vi "Todas_Coincidencias_3_detectores.vi"() -> ()   [LabVIEW 2010]
uses:
  <vilib>/Instr/_visa.llb/VISA Configure Serial Port (Instr).vi
  <vilib>/Utility/file.llb/Write To Spreadsheet File (string).vi
panel:
  in  "Esperando Cuentas":bool
  in  "# Ventanas\na correr":i32=1
  out "# Ventana\nactual":i32=1
  out "Finalizado":bool=TRUE
  in  "INICIAR":bool
  out "Listo":bool=TRUE
  out "Tiempo \nTranscurrido (s)":i32=1
  in  "Config_Tiempo":bool
  in  "Tiempo de la ventana":i32=100
  in  "Unidades de tiempo":u16(ring) items=["(x10)ns", "us", "ms"]
  in  "Error Bytes,":bool
  in  "Guardar":bool
  in  "file path (dialog if empty)":path
  out "D123":u64=5
  out "D3":u64=1
  out "D2":u64=5
  out "D1":u64=10
  out "D23":u64=3
  out "D13":u64=5
  out "D12":u64=10
  out "Lectura":string
  in  "stop":bool
  out "Error":errorcluster
  in  "Puerto USB":refnum<visa-resource-name>="COM20"
  # "Unidad de conteo de coincidencias"
  # "johny.jaramillo@udea.edu.co"
  # "daniel.estrada1@udea.edu.co"
  # "Coincidencia \ntriple"
  # "Detectores \nIndividuales"
  # "Coincidencias \ndobles"
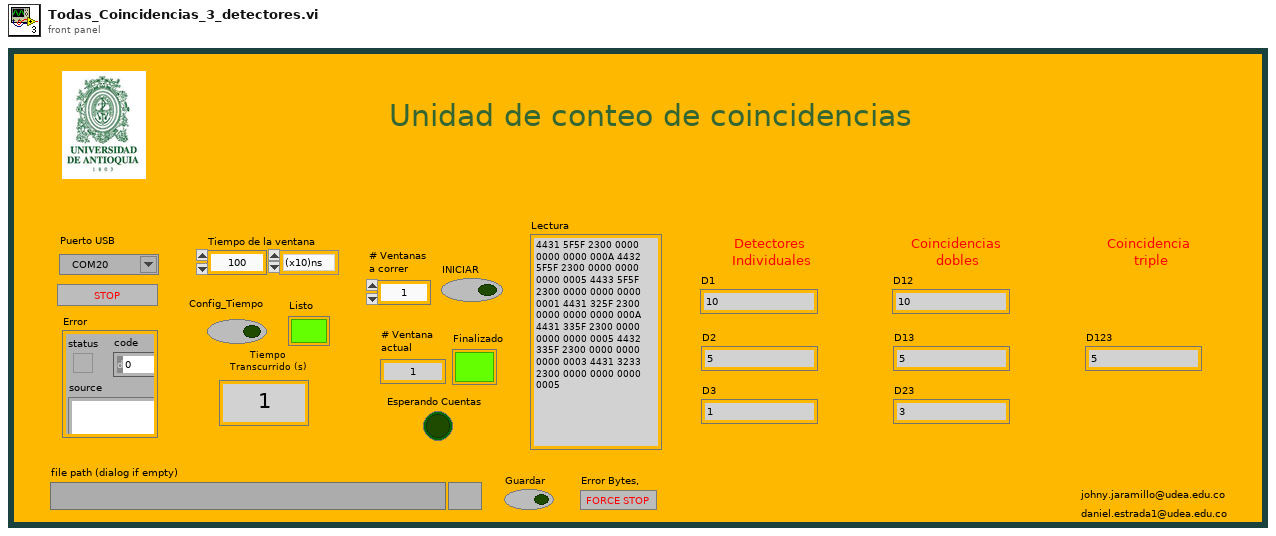
[diagram p1: front panel]
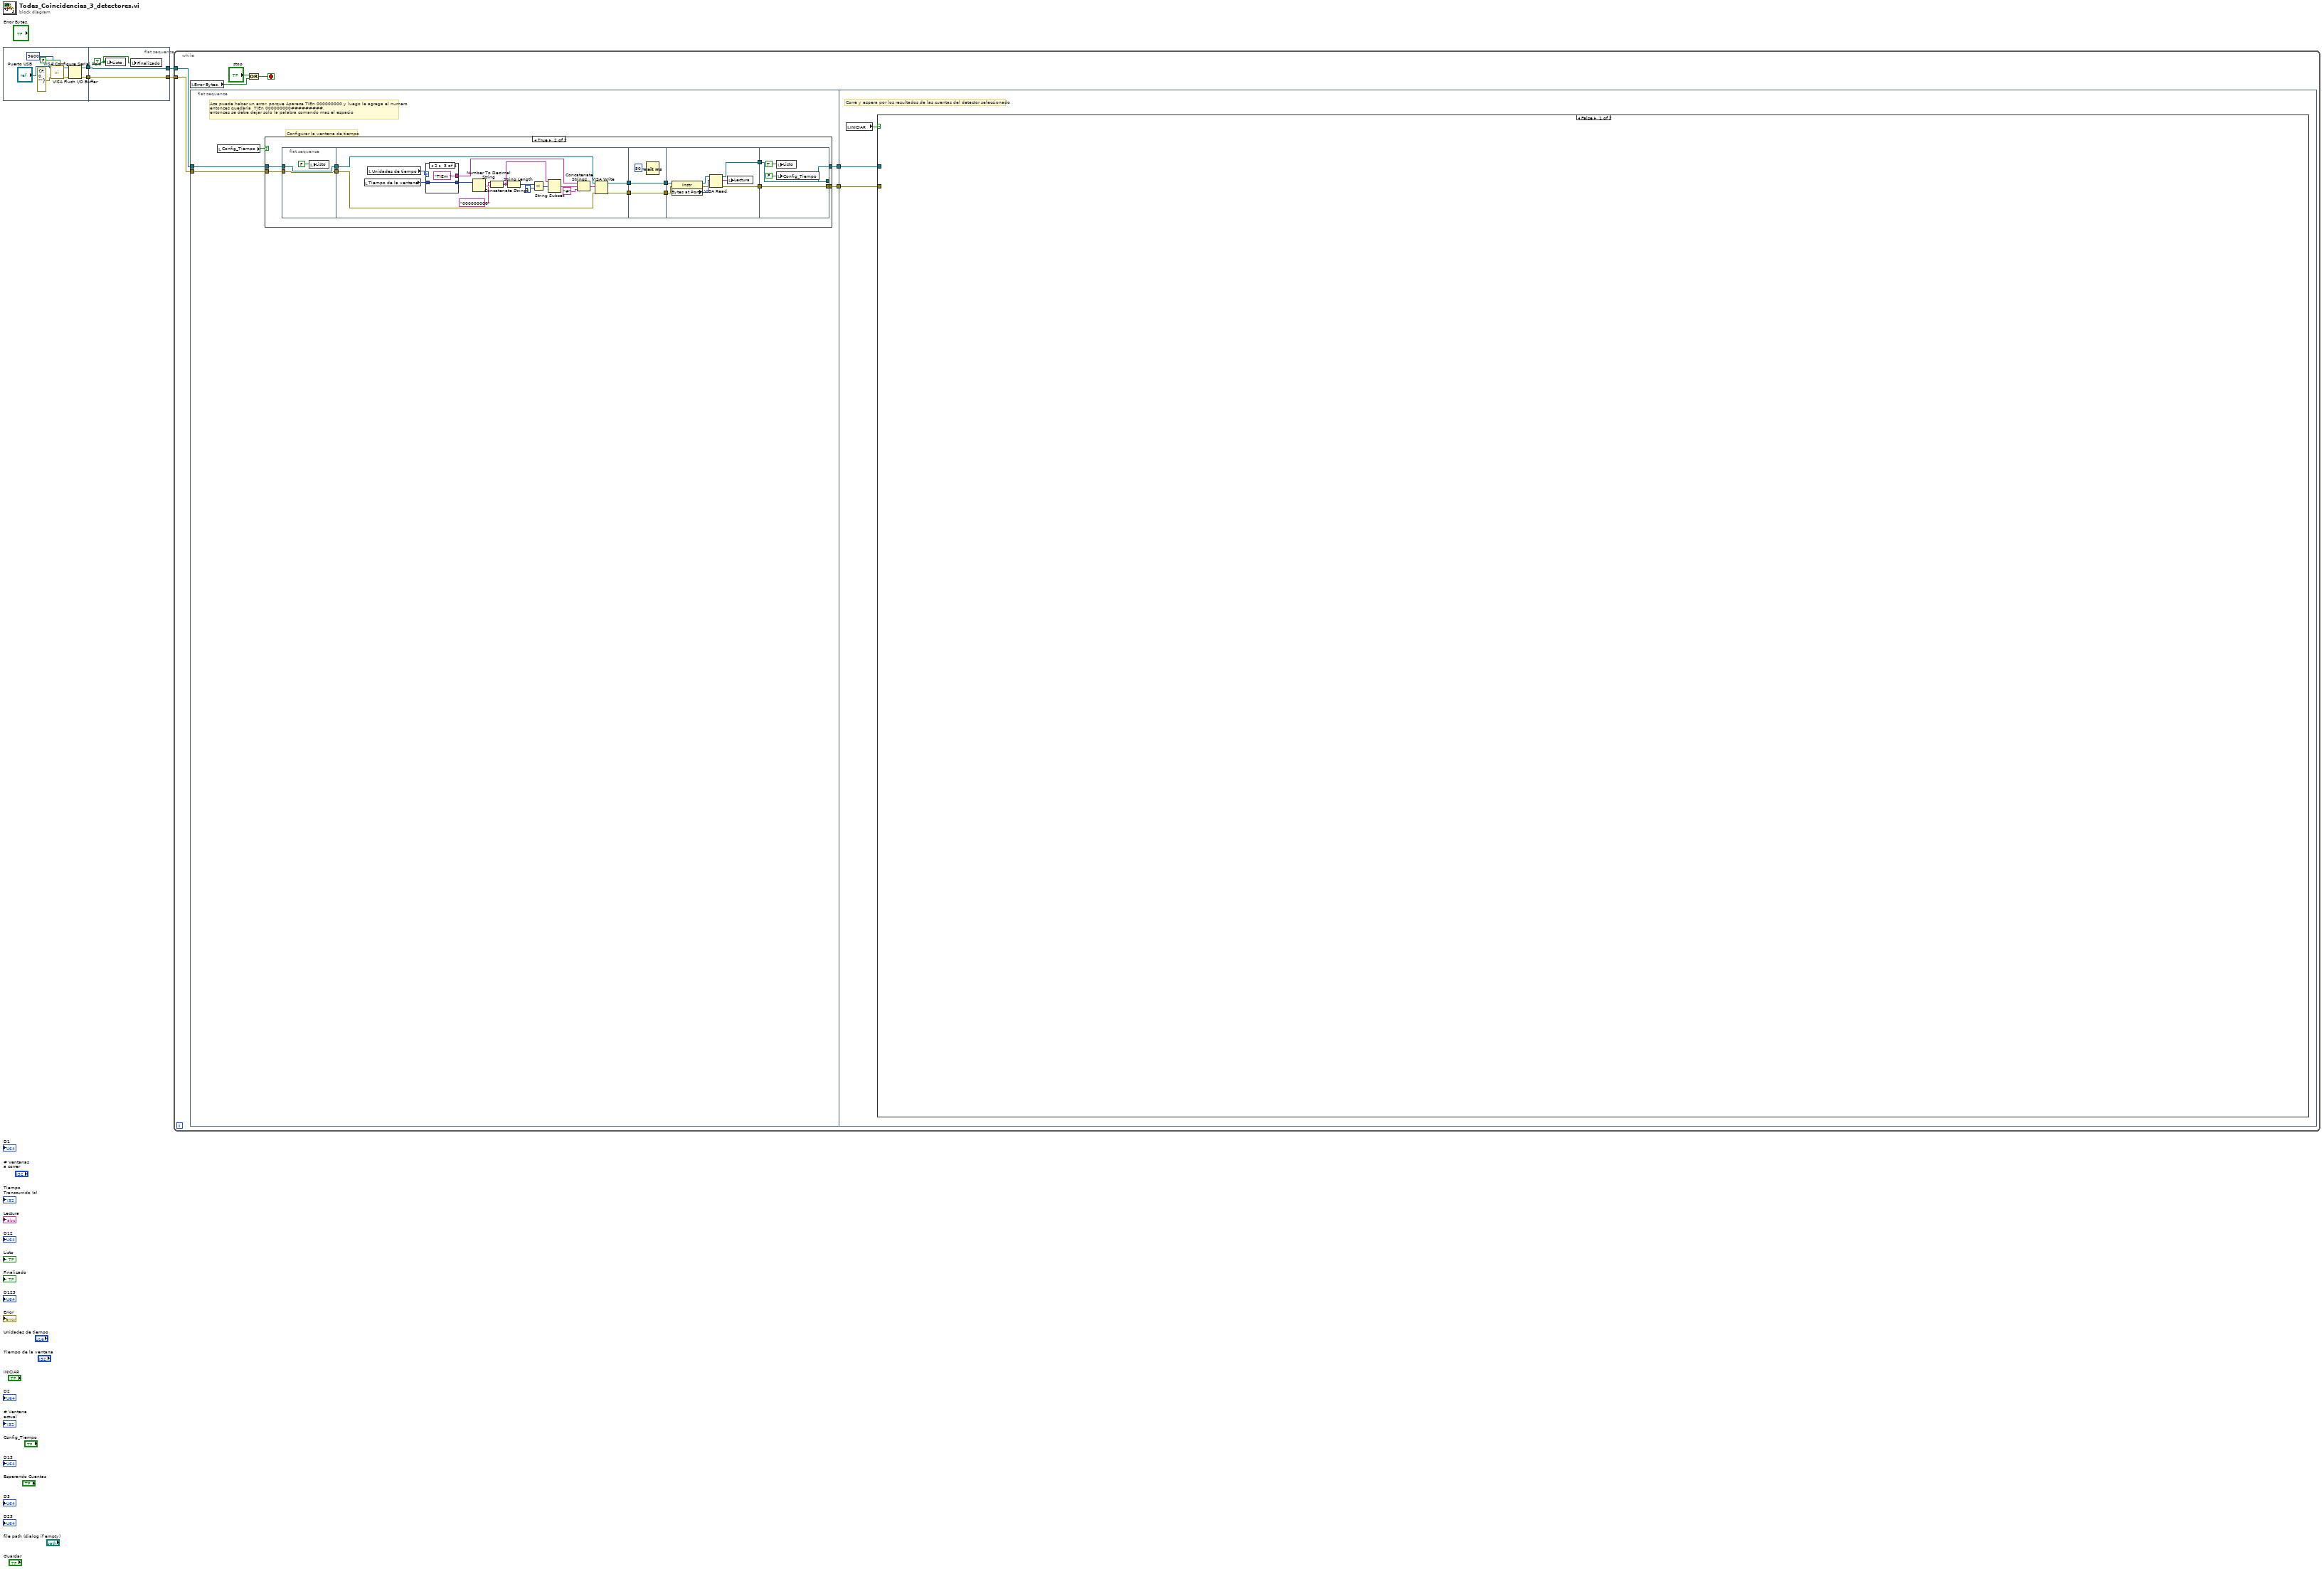
[diagram p0: block diagram]
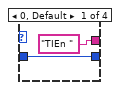
[diagram p3: hidden frame]
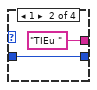
[diagram p4: hidden frame]
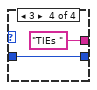
[diagram p5: hidden frame]
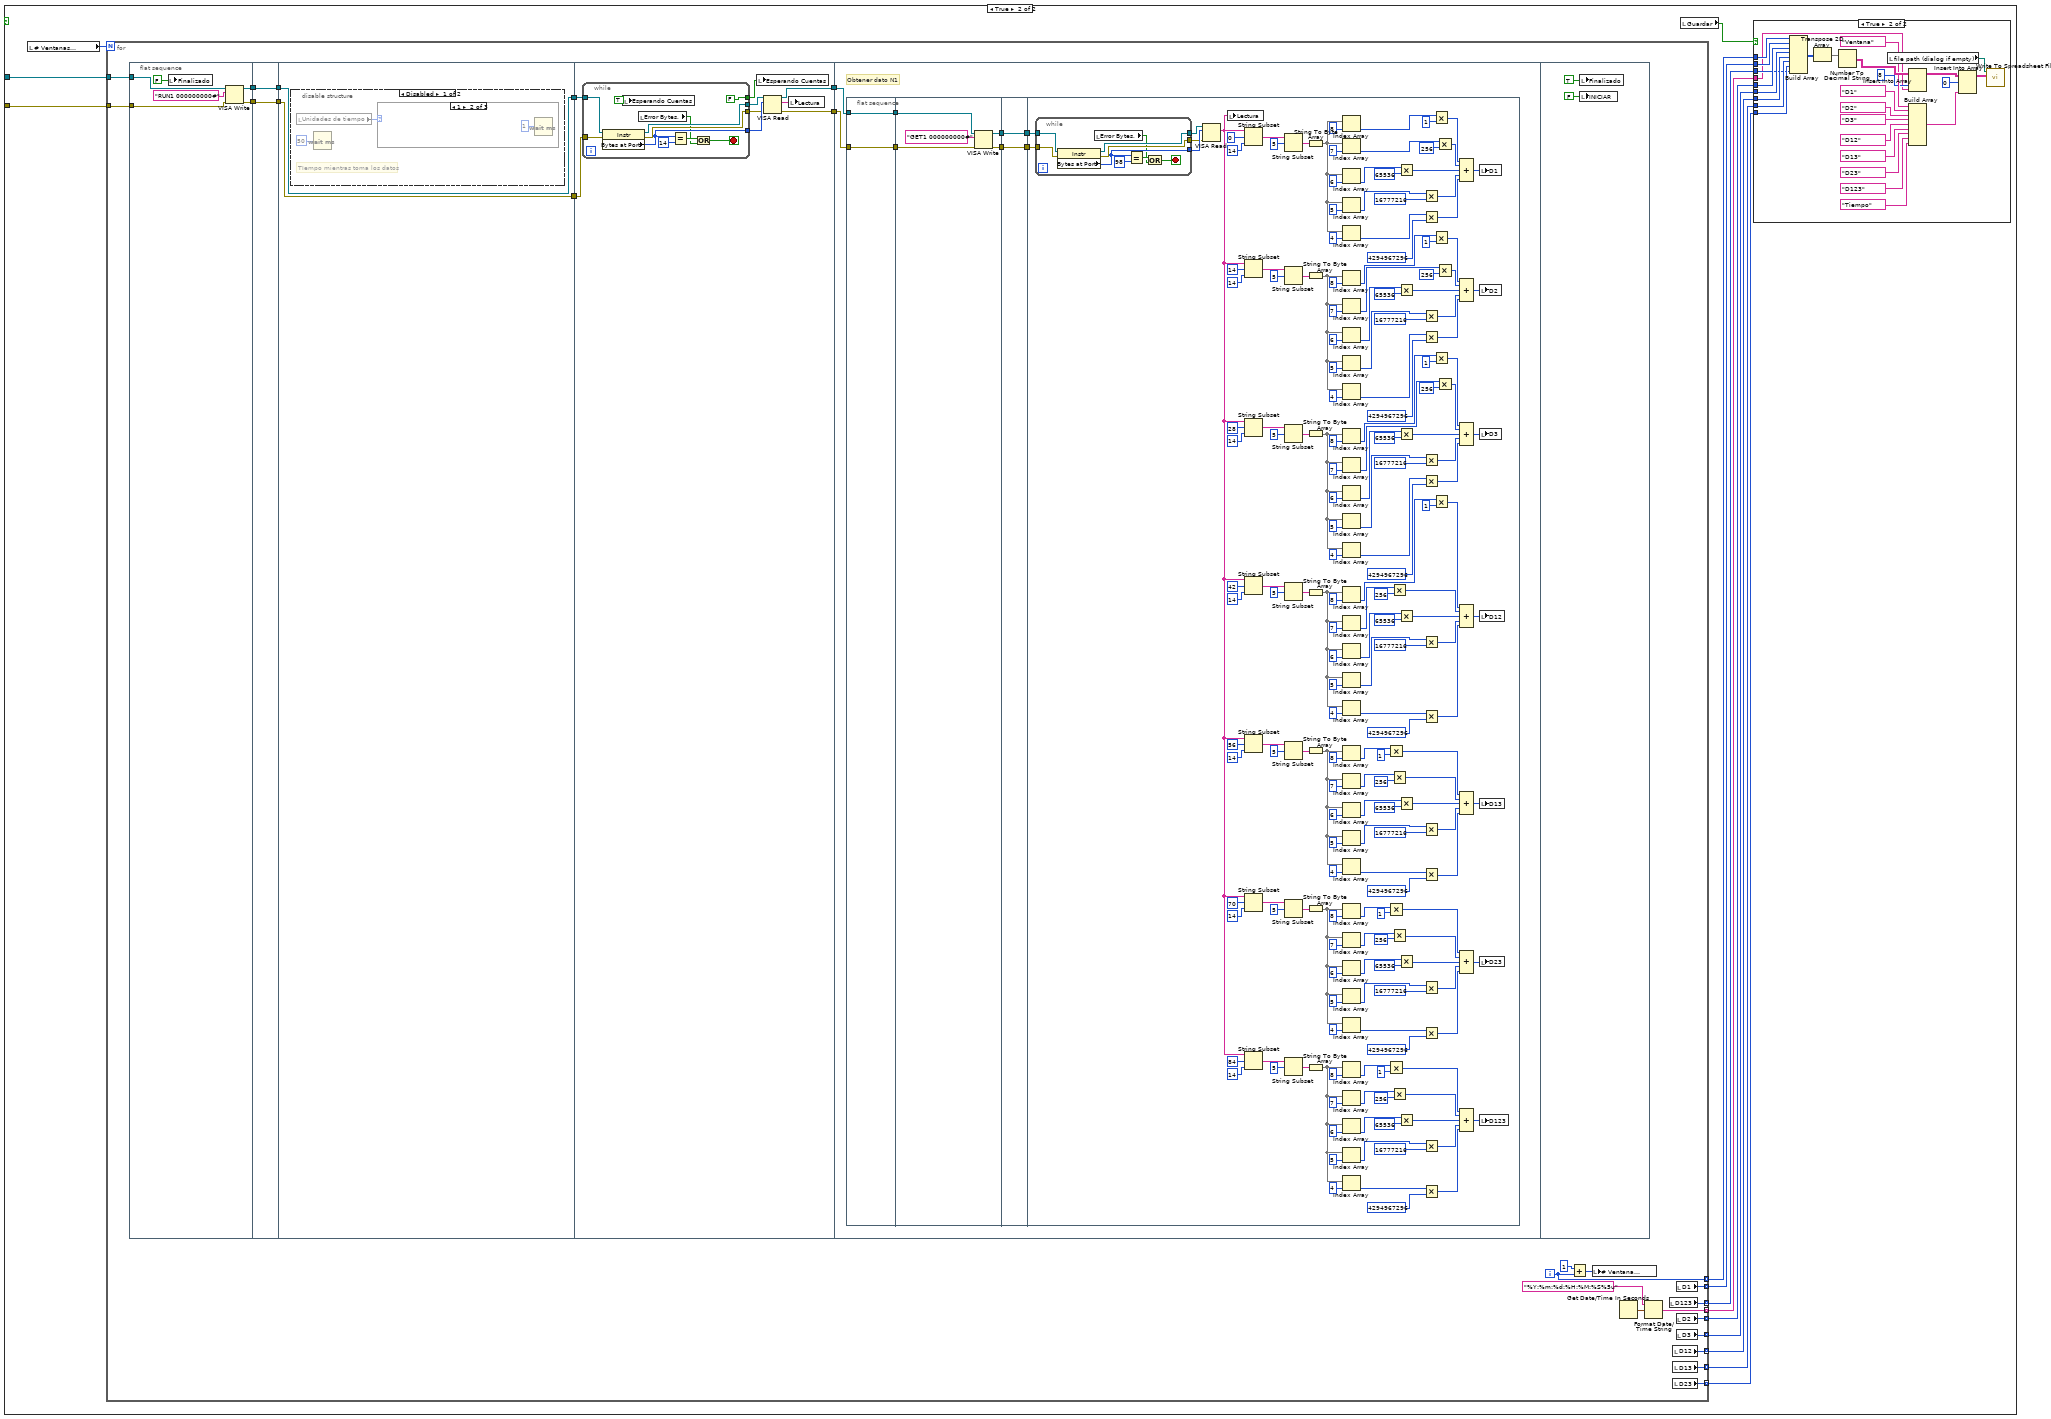
[diagram p6: hidden frame]
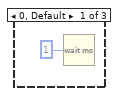
[diagram p8: hidden frame]
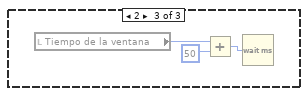
[diagram p9: hidden frame]
diagram:
  n1 = flat-sequence {
    tunnel: [w9] -> w4
    tunnel: [w8] -> w3
    tunnel: w4 -> [w14]
    tunnel: w3 -> [w13]
    tunnel: [w14] -> w2
    tunnel: [w13] -> w1
    frame #0 {
      n2 = call-poly "VISA Configure Serial Port"("VISA resource name"="Puerto USB", "Enable Termination\nChar (T)"=FALSE ("Enable Termination\nChar (T)"), "baud rate (9600)"=u32 9600, "error in (no error)"=errorcluster {"status"=FALSE, "code"=0, "source"=""}) -> ("VISA resource name out"=w7:refnum<visa-resource-name>, "error out"=w12:errorcluster)  [unwired: 10 in]
      n3 = VISA Flush I/O Buffer(VISA resource name=w7, error in (no error)=w12) -> (VISA resource name out=w9:refnum<visa-resource-name>, error out=w8:errorcluster)  [unwired: 1 in]
    }
    frame #1 {
      w15 = TRUE ("T. Done")
      n4 = local write "Listo"(w15) -> ()
      n5 = local write "Finalizado"(w15) -> ()
    }
  }
  n6 = while {
    tunnel: w2 -> [w20]
    tunnel: w1 -> [w19]
    stop <- w16 stop-if-true
    n7 = local read "Error Bytes,"() -> (w17:bool)
    n8 = flat-sequence {
      tunnel: [w26] -> w22
      tunnel: [w25] -> w21
      tunnel: w20 -> [w24]
      tunnel: w19 -> [w23]
      tunnel: w22 -> [w86]
      tunnel: w21 -> [w85]
      frame #0 {
        # "Aca puede haber un error, porque Aparece TIEn 000000000 y luego le agrega el numero\nentonces quedaria  TIEn 000000000#########,\nentonces se debe dejar solo la palabra comando mas el espacio"
        # "Configurar la ventana de tiempo"
        n9 = local read "Config_Tiempo"() -> (w27:bool)
        n10 = case shown="True" w27 {
          tunnel: [w29 w39] -> w26
          tunnel: [w28 w38] -> w25
          tunnel: w24 -> [w29 w41]
          tunnel: w23 -> [w28 w40]
          frame False {
          }
          frame True {
            n11 = flat-sequence {
              tunnel: w40 -> [w42]
              tunnel: w41 -> [w43]
              tunnel: [w43] -> w31
              tunnel: [w42] -> w30
              tunnel: [w59] -> w37
              tunnel: [w58] -> w35
              tunnel: w31 -> [w61]
              tunnel: w30 -> [w60]
              tunnel: w37 -> [w72]
              tunnel: [w72] -> w36
              tunnel: w35 -> [w71]
              tunnel: [w71] -> w34
              tunnel: w36 -> [w78]
              tunnel: w34 -> [w77]
              tunnel: [w75] -> w33
              tunnel: [w76] -> w32
              tunnel: [w83] -> w39
              tunnel: [w84] -> w38
              tunnel: w33 -> [w84]
              tunnel: w32 -> [w83]
              frame #0 {
                n12 = local write "Listo"(FALSE ("T. Done")) -> ()
              }
              frame #1 {
                n13 = local read "Tiempo de la ventana"() -> (w50:i32)
                n14 = local read "Unidades de tiempo"() -> (w51:u16)
                n15 = case shown="2" w51 {
                  tunnel: ["TIEn " ("string") "TIEu " ("string") "TIEm " ("string") "TIEs " ("string")] -> w57
                  tunnel: w50 -> [w62 w64 w66 w68]
                  tunnel: [w62 w64 w66 w68] -> w49
                  frame 0, Default {
                  }
                  frame 1 {
                  }
                  frame 2 {
                  }
                  frame 3 {
                  }
                }
                n16 = Number To Decimal String(number=w49) -> (decimal integer string=w53:string)  [unwired: 1 in]
                n17 = Concatenate Strings("000000000" ("string"), w53) -> (w54:string)
                n18 = String Length(string=w54) -> (length=w55:i32)
                n19 = Subtract(x=w55, y=9) -> (x-y=w46:i32)
                n20 = String Subset(string=w54, offset (0)=w46) -> (substring=w48:string)  [unwired: 1 in]
                n21 = Concatenate Strings(w57, w48, "#") -> (w45:string)
                n22 = VISA Write(VISA resource name=w61, write buffer=w45, error in (no error)=w60) -> (VISA resource name out=w59:refnum<visa-resource-name>, error out=w58:errorcluster)  [unwired: 1 out]
              }
              frame #2 {
                n23 = Wait (ms)(milliseconds to wait=u32 50) -> ()  [unwired: 1 out]
              }
              frame #3 {
                n24 = property class="Instr"(reference=w78, error in=w77) -> (reference out=w80:refnum<visa-resource-name>, error out=w74:errorcluster, "Bytes at Port"=w79:u32)
                n25 = VISA Read(VISA resource name=w80, byte count=w79, error in (no error)=w74) -> (VISA resource name out=w76:refnum<visa-resource-name>, read buffer=w73:string, error out=w75:errorcluster)  [unwired: 1 out]
                n26 = local write "Lectura"(w73) -> ()
              }
              frame #4 {
                n27 = local write "Listo"(TRUE ("T. Done")) -> ()
                n28 = local write "Config_Tiempo"(FALSE ("Config_Módulo")) -> ()
              }
            }
          }
        }
      }
      frame #1 {
        # "Corre y espera por los resultados de las cuentas del detector seleccionado"
        n29 = local read "INICIAR"() -> (w87:bool)
        n30 = case shown="False" w87 {
          tunnel: w86 -> [_ w100]
          tunnel: w85 -> [_ w99]
          frame False {
          }
          frame True {
            n31 = local read "# Ventanas\na correr"() -> (w98:i32)
            n32 = for {
              N: w98 -> [_]
              tunnel: w100 -> [w146]
              tunnel: w99 -> [w145]
              tunnel: [w137] -> w96 mode=indexing
              tunnel: [w144] -> w95 mode=indexing
              tunnel: [w143] -> w94 mode=indexing
              tunnel: [w142] -> w93 mode=indexing
              tunnel: [w141] -> w92 mode=indexing
              tunnel: [w140] -> w91 mode=indexing
              tunnel: [w139] -> w90 mode=indexing
              tunnel: [w138] -> w89 mode=indexing
              tunnel: [w129] -> w88 mode=indexing
              i -> [w137]
              n33 = flat-sequence {
                tunnel: w145 -> [w154]
                tunnel: w146 -> [w155]
                tunnel: [w153] -> w150
                tunnel: [w152] -> w149
                tunnel: w150 -> [w158]
                tunnel: [w158] -> w134
                tunnel: w149 -> [w157]
                tunnel: [w157] -> w132
                tunnel: w134 -> [w160]
                tunnel: [w160] -> w133
                tunnel: w132 -> [w159]
                tunnel: [w159] -> w131
                tunnel: [w169] -> w148
                tunnel: [w170] -> w147
                tunnel: w131 -> [w172]
                tunnel: w133 -> [w173]
                tunnel: w148 -> [w190]
                tunnel: w147 -> [w191]
                frame #0 {
                  n34 = local write "Finalizado"(FALSE ("Listo")) -> ()
                  n35 = VISA Write(VISA resource name=w155, write buffer="RUN1 000000000#", error in (no error)=w154) -> (VISA resource name out=w153:refnum<visa-resource-name>, error out=w152:errorcluster)  [unwired: 1 out]
                }
                frame #1 {
                }
                frame #2 {
                  n36 = disable-structure shown="Disabled" {
                    frame Disabled {
                      # "TIempo mientras toma los datos"
                      n37 = local read "Unidades de tiempo"() -> (w162:u16)
                      n38 = Wait (ms)(milliseconds to wait=u32 50) -> ()  [unwired: 1 out]
                      n39 = case shown="1" w162 {
                        frame 0, Default {
                          n40 = Wait (ms)(milliseconds to wait=u32 1) -> ()  [unwired: 1 out]
                        }
                        frame 1 {
                          n41 = Wait (ms)(milliseconds to wait=u32 1) -> ()  [unwired: 1 out]
                        }
                        frame 2 {
                          n42 = local read "Tiempo de la ventana"() -> (w167:i32)
                          n43 = Add(x=w167, y=50) -> (x+y=w166:i32)
                          n44 = Wait (ms)(milliseconds to wait=w166) -> ()  [unwired: 1 out]
                        }
                      }
                    }
                    frame Enabled {
                    }
                  }
                }
                frame #3 {
                  n45 = while {
                    tunnel: [w187] -> w176
                    tunnel: [w183] -> w175
                    tunnel: [w186] -> w174
                    tunnel: w173 -> [w185]
                    tunnel: w172 -> [w184]
                    tunnel: [FALSE ("esperando run")] -> w168
                    stop <- w179 stop-if-true
                    n46 = property class="Instr"(reference=w185, error in=w184) -> (reference out=w187:refnum<visa-resource-name>, error out=w186:errorcluster, "Bytes at Port"=w183:u32)
                    n47 = local write "Esperando Cuentas"(TRUE ("esperando run")) -> ()
                    n48 = local read "Error Bytes,"() -> (w180:bool)
                    n49 = Equal?(x=w183, y=u32 14) -> (x = y?=w181:bool)
                    n50 = Or(x=w181, y=w180) -> (x .or. y?=w179:bool)
                  }
                  n51 = local write "Esperando Cuentas"(w168) -> ()
                  n52 = VISA Read(VISA resource name=w176, byte count=w175, error in (no error)=w174) -> (VISA resource name out=w170:refnum<visa-resource-name>, read buffer=w171:string, error out=w169:errorcluster)  [unwired: 1 out]
                  n53 = local write "Lectura"(w171) -> ()
                }
                frame #4 {
                  # "Obtener dato N1"
                  n54 = flat-sequence {
                    tunnel: w190 -> [w196]
                    tunnel: w191 -> [w197]
                    tunnel: [w197] -> w189
                    tunnel: [w196] -> w188
                    tunnel: [w201] -> w195
                    tunnel: [w200] -> w194
                    tunnel: w189 -> [w199]
                    tunnel: w188 -> [w198]
                    tunnel: w195 -> [w204]
                    tunnel: w194 -> [w203]
                    tunnel: [w204] -> w193
                    tunnel: [w203] -> w192
                    tunnel: w193 -> [w372]
                    tunnel: w192 -> [w373]
                    frame #0 {
                    }
                    frame #1 {
                      n55 = VISA Write(VISA resource name=w199, write buffer="GET1 000000000#", error in (no error)=w198) -> (VISA resource name out=w200:refnum<visa-resource-name>, error out=w201:errorcluster)  [unwired: 1 out]
                    }
                    frame #2 {
                    }
                    frame #3 {
                      n56 = while {
                        tunnel: [w408] -> w376
                        tunnel: [w401] -> w375
                        tunnel: [w407] -> w374
                        tunnel: w373 -> [w406]
                        tunnel: w372 -> [w405]
                        stop <- w404 stop-if-true
                        n57 = property class="Instr"(reference=w406, error in=w405) -> (reference out=w408:refnum<visa-resource-name>, error out=w407:errorcluster, "Bytes at Port"=w401:u32)
                        n58 = local read "Error Bytes,"() -> (w400:bool)
                        n59 = Equal?(x=w401, y=u32 98) -> (x = y?=w403:bool)
                        n60 = Or(x=w403, y=w400) -> (x .or. y?=w404:bool)
                      }
                      n61 = VISA Read(VISA resource name=w376, byte count=w375, error in (no error)=w374) -> (read buffer=w205:string)  [unwired: 3 out]
                      n62 = local write "Lectura"(w205) -> ()
                      n63 = String Subset(string=w205, offset (0)=0, length (rest)=14 ("length (rest)")) -> (substring=w334:string)
                      n64 = String Subset(string=w205, offset (0)=14, length (rest)=14 ("length (rest)")) -> (substring=w215:string)
                      n65 = String Subset(string=w205, offset (0)=28, length (rest)=14 ("length (rest)")) -> (substring=w218:string)
                      n66 = String Subset(string=w205, offset (0)=42, length (rest)=14 ("length (rest)")) -> (substring=w214:string)
                      n67 = String Subset(string=w205, offset (0)=56, length (rest)=14 ("length (rest)")) -> (substring=w217:string)
                      n68 = String Subset(string=w205, offset (0)=70, length (rest)=14 ("length (rest)")) -> (substring=w213:string)
                      n69 = String Subset(string=w205, offset (0)=84, length (rest)=14 ("length (rest)")) -> (substring=w216:string)
                      n70 = String Subset(string=w334, offset (0)=5) -> (substring=w378:string)  [unwired: 1 in]
                      n71 = String Subset(string=w215, offset (0)=5) -> (substring=w266:string)  [unwired: 1 in]
                      n72 = String Subset(string=w218, offset (0)=5) -> (substring=w338:string)  [unwired: 1 in]
                      n73 = String Subset(string=w214, offset (0)=5) -> (substring=w243:string)  [unwired: 1 in]
                      n74 = String Subset(string=w217, offset (0)=5) -> (substring=w312:string)  [unwired: 1 in]
                      n75 = String Subset(string=w213, offset (0)=5) -> (substring=w220:string)  [unwired: 1 in]
                      n76 = String Subset(string=w216, offset (0)=5) -> (substring=w289:string)  [unwired: 1 in]
                      n77 = String To Byte Array(string=w378) -> (unsigned byte array=w399:u8[])
                      n78 = String To Byte Array(string=w266) -> (unsigned byte array=w287:u8[])
                      n79 = String To Byte Array(string=w338) -> (unsigned byte array=w359:u8[])
                      n80 = String To Byte Array(string=w243) -> (unsigned byte array=w264:u8[])
                      n81 = String To Byte Array(string=w312) -> (unsigned byte array=w333:u8[])
                      n82 = String To Byte Array(string=w220) -> (unsigned byte array=w241:u8[])
                      n83 = String To Byte Array(string=w289) -> (unsigned byte array=w310:u8[])
                      n84 = Index Array(array=w399, index=8) -> (element=w384:u8)
                      n85 = Index Array(array=w399, index=7) -> (element=w387:u8)
                      n86 = Index Array(array=w399, index=6) -> (element=w389:u8)
                      n87 = Index Array(array=w399, index=5) -> (element=w392:u8)
                      n88 = Index Array(array=w399, index=4) -> (element=w393:u8)
                      n89 = Index Array(array=w287, index=8) -> (element=w272:u8)
                      n90 = Index Array(array=w287, index=7) -> (element=w275:u8)
                      n91 = Index Array(array=w287, index=6) -> (element=w277:u8)
                      n92 = Index Array(array=w287, index=5) -> (element=w280:u8)
                      n93 = Index Array(array=w287, index=4) -> (element=w281:u8)
                      n94 = Index Array(array=w359, index=8) -> (element=w344:u8)
                      n95 = Index Array(array=w359, index=7) -> (element=w347:u8)
                      n96 = Index Array(array=w359, index=6) -> (element=w349:u8)
                      n97 = Index Array(array=w359, index=5) -> (element=w352:u8)
                      n98 = Index Array(array=w359, index=4) -> (element=w353:u8)
                      n99 = Index Array(array=w264, index=8) -> (element=w249:u8)
                      n100 = Index Array(array=w264, index=7) -> (element=w252:u8)
                      n101 = Index Array(array=w264, index=6) -> (element=w254:u8)
                      n102 = Index Array(array=w264, index=5) -> (element=w257:u8)
                      n103 = Index Array(array=w264, index=4) -> (element=w258:u8)
                      n104 = Index Array(array=w333, index=8) -> (element=w318:u8)
                      n105 = Index Array(array=w333, index=7) -> (element=w321:u8)
                      n106 = Index Array(array=w333, index=6) -> (element=w323:u8)
                      n107 = Index Array(array=w333, index=5) -> (element=w326:u8)
                      n108 = Index Array(array=w333, index=4) -> (element=w327:u8)
                      n109 = Index Array(array=w241, index=8) -> (element=w226:u8)
                      n110 = Index Array(array=w241, index=7) -> (element=w229:u8)
                      n111 = Index Array(array=w241, index=6) -> (element=w231:u8)
                      n112 = Index Array(array=w241, index=5) -> (element=w234:u8)
                      n113 = Index Array(array=w241, index=4) -> (element=w235:u8)
                      n114 = Index Array(array=w310, index=8) -> (element=w295:u8)
                      n115 = Index Array(array=w310, index=7) -> (element=w298:u8)
                      n116 = Index Array(array=w310, index=6) -> (element=w300:u8)
                      n117 = Index Array(array=w310, index=5) -> (element=w303:u8)
                      n118 = Index Array(array=w310, index=4) -> (element=w304:u8)
                      n119 = Multiply(x=w318, y=u64 1) -> (x*y=w328:u64)
                      n120 = Multiply(x=w226, y=u64 1) -> (x*y=w236:u64)
                      n121 = Multiply(x=w295, y=u64 1) -> (x*y=w305:u64)
                      n122 = Multiply(x=w252, y=u64 256) -> (x*y=w260:u64)
                      n123 = Multiply(x=w321, y=u64 256) -> (x*y=w329:u64)
                      n124 = Multiply(x=w229, y=u64 256) -> (x*y=w237:u64)
                      n125 = Multiply(x=w298, y=u64 256) -> (x*y=w306:u64)
                      n126 = Multiply(x=w389, y=u64 65536) -> (x*y=w396:u64)
                      n127 = Multiply(x=w277, y=u64 65536) -> (x*y=w284:u64)
                      n128 = Multiply(x=w349, y=u64 65536) -> (x*y=w356:u64)
                      n129 = Multiply(x=w254, y=u64 65536) -> (x*y=w261:u64)
                      n130 = Multiply(x=w323, y=u64 65536) -> (x*y=w330:u64)
                      n131 = Multiply(x=w231, y=u64 65536) -> (x*y=w238:u64)
                      n132 = Multiply(x=w300, y=u64 65536) -> (x*y=w307:u64)
                      n133 = Multiply(x=w392, y=u64 16777216) -> (x*y=w397:u64)
                      n134 = Multiply(x=w393, y=u64 4294967296) -> (x*y=w398:u64)
                      n135 = Multiply(x=w280, y=u64 16777216) -> (x*y=w285:u64)
                      n136 = Multiply(x=w281, y=u64 4294967296) -> (x*y=w286:u64)
                      n137 = Multiply(x=w352, y=u64 16777216) -> (x*y=w357:u64)
                      n138 = Multiply(x=w353, y=u64 4294967296) -> (x*y=w358:u64)
                      n139 = Multiply(x=w257, y=u64 16777216) -> (x*y=w262:u64)
                      n140 = Multiply(x=w258, y=u64 4294967296) -> (x*y=w263:u64)
                      n141 = Multiply(x=w326, y=u64 16777216) -> (x*y=w331:u64)
                      n142 = Multiply(x=w327, y=u64 4294967296) -> (x*y=w332:u64)
                      n143 = Multiply(x=w234, y=u64 16777216) -> (x*y=w239:u64)
                      n144 = Multiply(x=w235, y=u64 4294967296) -> (x*y=w240:u64)
                      n145 = Multiply(x=w303, y=u64 16777216) -> (x*y=w308:u64)
                      n146 = Multiply(x=w304, y=u64 4294967296) -> (x*y=w309:u64)
                      n147 = Multiply(x=w384, y=u64 1) -> (x*y=w394:u64)
                      n148 = Multiply(x=w272, y=u64 1) -> (x*y=w282:u64)
                      n149 = Multiply(x=w344, y=u64 1) -> (x*y=w354:u64)
                      n150 = Multiply(x=w249, y=u64 1) -> (x*y=w259:u64)
                      n151 = Multiply(x=w387, y=u64 256) -> (x*y=w395:u64)
                      n152 = Multiply(x=w275, y=u64 256) -> (x*y=w283:u64)
                      n153 = Multiply(x=w347, y=u64 256) -> (x*y=w355:u64)
                      n154 = Compound Arithmetic op=ADD(w394, w395, w396, w397, w398) -> (w212:u64)
                      n155 = Compound Arithmetic op=ADD(w282, w283, w284, w285, w286) -> (w206:u64)
                      n156 = Compound Arithmetic op=ADD(w354, w355, w356, w357, w358) -> (w211:u64)
                      n157 = Compound Arithmetic op=ADD(w259, w260, w261, w262, w263) -> (w207:u64)
                      n158 = Compound Arithmetic op=ADD(w328, w329, w330, w331, w332) -> (w210:u64)
                      n159 = Compound Arithmetic op=ADD(w236, w237, w238, w239, w240) -> (w208:u64)
                      n160 = Compound Arithmetic op=ADD(w305, w306, w307, w308, w309) -> (w209:u64)
                      n161 = local write "D1"(w212) -> ()
                      n162 = local write "D2"(w206) -> ()
                      n163 = local write "D3"(w211) -> ()
                      n164 = local write "D12"(w207) -> ()
                      n165 = local write "D13"(w210) -> ()
                      n166 = local write "D23"(w208) -> ()
                      n167 = local write "D123"(w209) -> ()
                    }
                  }
                }
                frame #5 {
                  n168 = local write "Finalizado"(TRUE ("Listo")) -> ()
                  n169 = local write "INICIAR"(FALSE ("Config_Módulo")) -> ()
                }
              }
              n170 = Add(x=1, y=w137) -> (x+y=w135:i32)
              n171 = local write "# Ventana\nactual"(w135) -> ()
              n172 = Get Date/Time In Seconds() -> (seconds since 1Jan1904=w130:timestamp)
              n173 = Format Date/Time String(time format string (%c)="%Y:%m:%d:%H:%M:%S%5u", seconds (now)=w130) -> (date/time string=w129:string)  [unwired: 1 in]
              n174 = local read "D123"() -> (w138:u64)
              n175 = local read "D12"() -> (w141:u64)
              n176 = local read "D13"() -> (w140:u64)
              n177 = local read "D23"() -> (w139:u64)
              n178 = local read "D1"() -> (w144:u64)
              n179 = local read "D2"() -> (w143:u64)
              n180 = local read "D3"() -> (w142:u64)
            }
            n181 = local read "Guardar"() -> (w97:bool)
            n182 = case shown="True" w97 {
              tunnel: w95 -> [_ w126]
              tunnel: w96 -> [_ w125]
              tunnel: w94 -> [_ w124]
              tunnel: w93 -> [_ w123]
              tunnel: w92 -> [_ w122]
              tunnel: w91 -> [_ w121]
              tunnel: w90 -> [_ w120]
              tunnel: w89 -> [_ w119]
              tunnel: w88 -> [_ w102]
              frame False {
              }
              frame True {
                n183 = Build Array(w125, w126, w124, w123, w122, w121, w120, w119) -> (w108:u64[][])
                n184 = Transpose 2D Array(2D array=w108) -> (transposed array=w107:u64[][])
                n185 = Number To Decimal String(number=w107) -> (decimal integer string=w118:string[][])  [unwired: 1 in]
                n186 = local read "file path (dialog if empty)"() -> (w127:path)
                n187 = Insert Into Array(array=w118, index (col)=8 ("index (row)"), new element=w102) -> (w106:string[][])  [unwired: 1 in]
                n188 = Build Array("Ventana", "D1", "D2", "D3", "D12", "D13", "D23", "D123", "Tiempo") -> (w101:string[])
                n189 = Insert Into Array(array=w106, index (row)=0 ("disabled index (col)"), new element=w101) -> (w105:string[][])  [unwired: 1 in]
                n190 = call-poly <vilib>:"Write To Spreadsheet File.vi"("2D data"=w105, "file path (dialog if empty)"=w127) -> ()  [unwired: 6 in, 1 out]
              }
            }
          }
        }
      }
    }
    n191 = Or(x="stop", y=w17) -> (x .or. y?=w16:bool)
  }
